vi "ML AI Player.vi"(0 "Total Player number":i32, 1 "Current Player ID number":i32, 2 "queue output":refnum<queue>, 3 "queue input":refnum<queue>) -> ()   [LabVIEW 2021]
uses:
  <vilib>/Utility/file.llb/Read Delimited Spreadsheet (DBL).vi
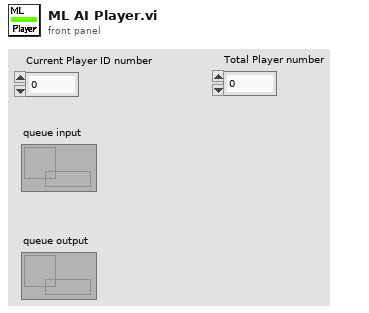
[diagram p1: front panel]
types:
  T1 = cluster{"all rows[1]":dbl, "all rows[2]":dbl, "all rows[3]":dbl, "all rows[4]":dbl, "all rows[5]":dbl, "all rows[6]":dbl, "all rows[7]":dbl, "all rows[8]":dbl, "all rows[9]":dbl}[]
  T2 = cluster{"X":dbl, "Y":dbl, "Object type":dbl, "Radius":dbl, "Width":dbl, "Height":dbl, "Theta":dbl, "HP":dbl, "R":dbl, "G":dbl, "B":dbl}[]
  T3 = cluster{"all rows[0]":dbl, "all rows[1]":dbl, "all rows[2]":dbl, "all rows[3]":dbl, "all rows[4]":dbl, "all rows[5]":dbl, "all rows[6]":dbl, "all rows[7]":dbl, "all rows[8]":dbl, "all rows[9]":dbl}
  T4 = cluster{"all rows[1]":dbl, "all rows[2]":dbl, "all rows[3]":dbl, "all rows[4]":dbl, "all rows[5]":dbl, "all rows[6]":dbl, "all rows[7]":dbl, "all rows[8]":dbl, "all rows[9]":dbl}
  T5 = cluster{"X":dbl, "Y":dbl, "Object type":dbl, "Radius":dbl, "Width":dbl, "Height":dbl, "Theta":dbl, "HP":dbl, "R":dbl, "G":dbl, "B":dbl}
  T6 = cluster{"D1":dbl, "D2":dbl, "D3":dbl, "D4":dbl, "D5":dbl, "D6":dbl, "D7":dbl, "D8":dbl}
  T7 = cluster{"Theta (toward that target)":dbl, "Distance (toward that target)":dbl, "Reachable":bool}
  T8 = cluster{dbl, dbl, "y":dbl, "y":dbl, "y":dbl, "y":dbl}
  T9 = cluster{dbl, dbl, "Theta (toward that target)":dbl, "f":dbl}
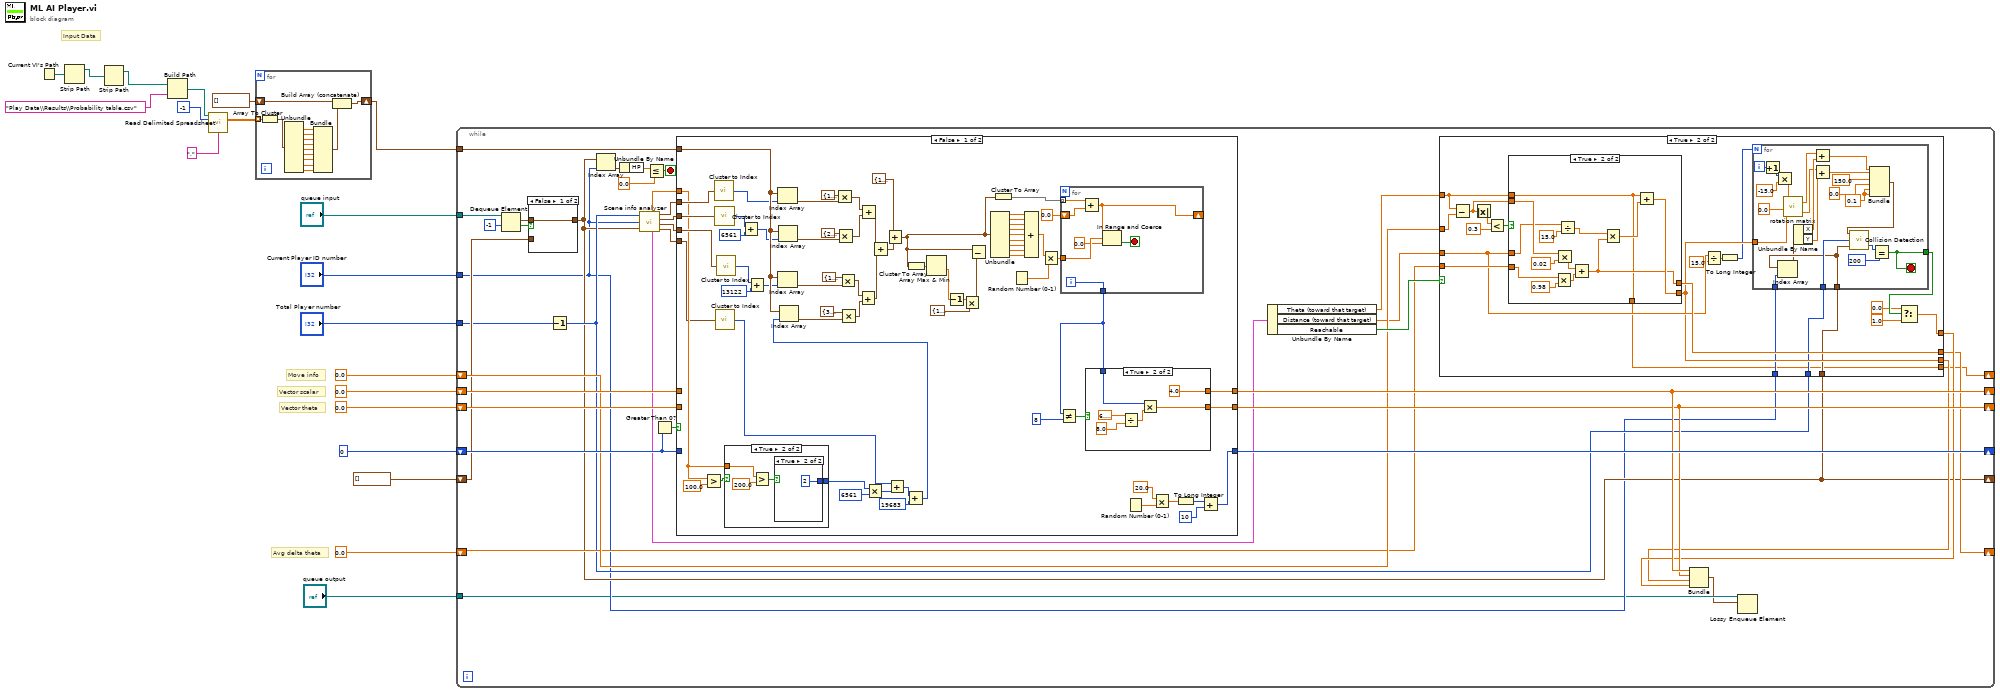
[diagram p0: block diagram]
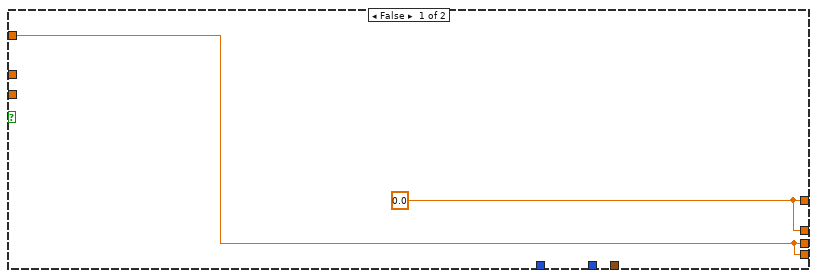
[diagram p3: hidden frame]
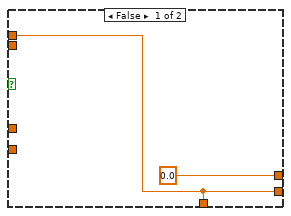
[diagram p4: hidden frame]
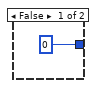
[diagram p5: hidden frame]
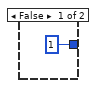
[diagram p6: hidden frame]
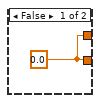
[diagram p7: hidden frame]
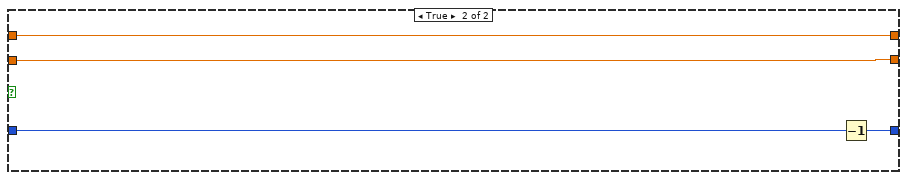
[diagram p8: hidden frame]
diagram:
  # "Input Data"
  # "Avg delta theta"
  # "Vector theta"
  # "Vector scalar"
  # "Move info"
  n1 = Current VI's Path() -> (path=w7:path)
  n2 = Strip Path(path=w7) -> (stripped path=w6:path)  [unwired: 1 out]
  n3 = Strip Path(path=w6) -> (stripped path=w5:path)  [unwired: 1 out]
  n4 = Build Path(base path=w5, name or relative path="Play Data\\Results\\Probability table.csv" ("delimiter (\\t)")) -> (appended path=w10:path)
  n5 = call-poly <vilib>:"Read Delimited Spreadsheet.vi"("file path (dialog if empty)"=w10, "number of rows (all:-1)"=-1, "delimiter (\\t)"="," ("delimiter (\\t)")) -> ("all rows"=w3:dbl[][])  [unwired: 7 in, 5 out]
  n6 = for {
    tunnel: w3 -> [w34] mode=indexing
    shift-right: [w33] -> w2
    shift-left: T1 [] -> [w32]
    n7 = Array To Cluster(array=w34) -> (cluster=w31:T3)
    n8 = Unbundle(w31) -> ("all rows[1]"=w30:dbl, "all rows[2]"=w29:dbl, "all rows[3]"=w28:dbl, "all rows[4]"=w27:dbl, "all rows[5]"=w26:dbl, "all rows[6]"=w25:dbl, "all rows[7]"=w24:dbl, "all rows[8]"=w23:dbl, "all rows[9]"=w22:dbl)  [unwired: 1 out]
    n9 = Bundle("all rows[1]"=w30, "all rows[2]"=w29, "all rows[3]"=w28, "all rows[4]"=w27, "all rows[5]"=w26, "all rows[6]"=w25, "all rows[7]"=w24, "all rows[8]"=w23, "all rows[9]"=w22) -> (w21:T4)  [unwired: 1 in]
    n10 = Build Array (concatenate)(w32, w21) -> (w33:T1)
  }
  n11 = while {
    tunnel: "queue input" -> [w41]
    shift-right: [w72] -> _
    shift-left: 0 -> [w70]
    tunnel: "queue output" -> [w37]
    shift-right: [w46] -> _
    shift-left: 0.0 -> [w58]
    shift-right: [w62] -> _
    shift-left: 0.0 -> [w64]
    shift-right: [w61] -> _
    shift-left: 0.0 -> [w63]
    shift-right: [w52] -> _
    shift-left: 0.0 -> [w53]
    shift-right: [w45] -> _
    shift-left: T2 [] ("Map Entity Object Position") -> [w44]
    tunnel: "Current Player ID number" -> [w43]
    tunnel: "Total Player number" -> [w42]
    tunnel: w2 -> [w35]
    stop <- w48 stop-if-true
    n12 = Dequeue Element(queue=w41, timeout in ms (-1)=-1) -> (element=w40:T2, timed out?=w38:bool)  [unwired: 1 in, 2 out]
    n13 = case shown="False" w38 {
      tunnel: [w73 w74] -> w45
      tunnel: w40 -> [w73 _]
      tunnel: w44 -> [_ w74]
      frame False {
      }
      frame True {
      }
    }
    n14 = Decrement(x=w42) -> (x-1=w51:i32)
    n15 = Index Array(array=w45, index=w43) -> (element=w50:T5)
    n16 = Unbundle By Name(w50) -> ("HP"=w49:dbl)
    n17 = call "Scene info analyzer.vi"("Map Entity Object Position"=w45, "Current Player ID"=w43, "Max Player ID"=w51) -> ("Enemy on 8 directions"=w65:T6, "Closest valid target"=w60:T7, "Farther Bullets on 8 directions"=w66:T6, "Closer Bullets on 8 directions"=w67:T6, "Current Player HP"=w69:dbl, "Object on 8 directions"=w68:T6)
    n18 = Less Or Equal?(x=w49, y=0.0) -> (x <= y?=w48:bool)
    n19 = Greater Than 0?(x=w70) -> (x > 0?=w71:bool)
    n20 = case shown="False" w71 {
      tunnel: [w203 w228] -> w72
      tunnel: w70 -> [_ w229]
      tunnel: w69 -> [w140 _]
      tunnel: w68 -> [w149 _]
      tunnel: w67 -> [w155 _]
      tunnel: w66 -> [w148 _]
      tunnel: w65 -> [w138 _]
      tunnel: w64 -> [_ w227]
      tunnel: w63 -> [_ w226]
      tunnel: [w204 w226] -> w61
      tunnel: [w166 w227] -> w62
      tunnel: w35 -> [w157 _]
      frame False {
        n21 = Greater?(x=w140, y=100.0) -> (0:w141:bool)
        n22 = call "Cluster to Index.vi"("Object on 8 directions"=w149) -> ("Index"=w156:i32)
        n23 = call "Cluster to Index.vi"("Object on 8 directions"=w155) -> ("Index"=w154:i32)
        n24 = call "Cluster to Index.vi"("Object on 8 directions"=w138) -> ("Index"=w137:i32)
        n25 = call "Cluster to Index.vi"("Object on 8 directions"=w148) -> ("Index"=w147:i32)
        n26 = case shown="True" w141 {
          tunnel: w140 -> [_ w207]
          tunnel: [0 ("y") w206] -> w139
          frame False {
          }
          frame True {
            n27 = Greater?(x=w207, y=200.0) -> (0:w208:bool)
            n28 = case shown="True" w208 {
              tunnel: [1 ("y") 2 ("y")] -> w206
              frame False {
              }
              frame True {
              }
            }
          }
        }
        n29 = Add(x=w154, y=6561) -> (x+y=w151:i32)
        n30 = Add(x=w147, y=13122) -> (x+y=w150:i32)
        n31 = Index Array(array=w157, index=w156) -> (element=w178:T4)
        n32 = Index Array(array=w157, index=w150) -> (element=w158:T4)
        n33 = Index Array(array=w157, index=w151) -> (element=w160:T4)
        n34 = Multiply(x=T4 {"all rows[1]"=1.5, "all rows[2]"=1.5, "all rows[3]"=1.5, "all rows[4]"=1.5, "all rows[5]"=1.5, "all rows[6]"=1.5, "all rows[7]"=1.5, "all rows[8]"=1.5, "all rows[9]"=1.5}, y=w178) -> (x*y=w179:T4)
        n35 = Multiply(x=T4 {"all rows[1]"=2.0, "all rows[2]"=2.0, "all rows[3]"=2.0, "all rows[4]"=2.0, "all rows[5]"=2.0, "all rows[6]"=2.0, "all rows[7]"=2.0, "all rows[8]"=2.0, "all rows[9]"=2.0}, y=w160) -> (x*y=w202:T4)
        n36 = Multiply(x=T4 {"all rows[1]"=1.5, "all rows[2]"=1.5, "all rows[3]"=1.5, "all rows[4]"=1.5, "all rows[5]"=1.5, "all rows[6]"=1.5, "all rows[7]"=1.5, "all rows[8]"=1.5, "all rows[9]"=1.5}, y=w158) -> (x*y=w201:T4)
        n37 = Add(x=w179, y=w202) -> (x+y=w199:T4)
        n38 = Multiply(x=w139, y=6561) -> (x*y=w143:i32)
        n39 = Add(x=w137, y=w143) -> (x+y=w145:i32)
        n40 = Add(x=w145, y=19683) -> (x+y=w136:i32)
        n41 = Index Array(array=w157, index=w136) -> (element=w159:T4)
        n42 = Multiply(x=T4 {"all rows[1]"=3.0, "all rows[2]"=3.0, "all rows[3]"=3.0, "all rows[4]"=3.0, "all rows[5]"=3.0, "all rows[6]"=3.0, "all rows[7]"=3.0, "all rows[8]"=3.0, "all rows[9]"=3.0}, y=w159) -> (x*y=w200:T4)
        n43 = Add(x=w201, y=w200) -> (x+y=w198:T4)
        n44 = Add(x=w199, y=w198) -> (x+y=w162:T4)
        n45 = Add(x=T4 {"all rows[1]"=1.0, "all rows[2]"=1.0, "all rows[3]"=1.0, "all rows[4]"=1.0, "all rows[5]"=1.0, "all rows[6]"=1.0, "all rows[7]"=1.0, "all rows[8]"=1.0, "all rows[9]"=1.0}, y=w162) -> (x+y=w161:T4)
        n46 = Cluster To Array(cluster=w161) -> (array=w172:dbl[])
        n47 = Array Max & Min(array=w172) -> (min value=w165:dbl)  [unwired: 3 out]
        n48 = Decrement(x=w165) -> (x-1=w164:dbl)
        n49 = Multiply(x=w164, y=T4 {"all rows[1]"=1.0, "all rows[2]"=1.0, "all rows[3]"=1.0, "all rows[4]"=1.0, "all rows[5]"=1.0, "all rows[6]"=1.0, "all rows[7]"=1.0, "all rows[8]"=1.0, "all rows[9]"=1.0} ("x")) -> (x*y=w170:T4)
        n50 = Subtract(x=w161, y=w170) -> ()  [unwired: 1 out]
        n51 = Unbundle(w161) -> ("all rows[1]"=w197:dbl, "all rows[2]"=w196:dbl, "all rows[3]"=w195:dbl, "all rows[4]"=w194:dbl, "all rows[5]"=w193:dbl, "all rows[6]"=w192:dbl, "all rows[7]"=w191:dbl, "all rows[8]"=w190:dbl, "all rows[9]"=w173:dbl)
        n52 = Cluster To Array(cluster=w161) -> (array=w187:dbl[])
        n53 = Random Number (0-1)() -> (number: 0 to 1=w189:dbl)
        n54 = Compound Arithmetic op=ADD(w197, w196, w195, w194, w193, w192, w191, w190, w173) -> (w188:dbl)
        n55 = Multiply(x=w188, y=w189) -> (x*y=w185:dbl)
        n56 = for {
          tunnel: w187 -> [w224] mode=indexing
          shift-right: [w223] -> _
          shift-left: 0.0 -> [w225]
          tunnel: w185 -> [w222]
          tunnel: [w221] -> w168
          i -> [w221]
          stop <- w220 stop-if-true
          n57 = Add(x=w224, y=w225) -> (x+y=w223:dbl)
          n58 = In Range and Coerce(upper limit=w223, x=w222, lower limit=0.0) -> (In Range?=w220:bool)  [unwired: 1 out]
        }
        n59 = Not Equal?(x=w168, y=8) -> (x != y?=w167:bool)
        n60 = case shown="True" w167 {
          tunnel: [w212 w218] -> w204
          tunnel: w168 -> [_ w214]
          tunnel: [w212 4.0] -> w166
          frame False {
            w212 = 0.0
          }
          frame True {
            n61 = Divide(x=6.283185307179586, y=8.0) -> (x/y=w215:dbl)
            n62 = Multiply(x=w214, y=w215) -> (x*y=w218:dbl)
          }
        }
        n63 = Random Number (0-1)() -> (number: 0 to 1=w183:dbl)
        n64 = Multiply(x=20.0, y=w183) -> (x*y=w182:dbl)
        n65 = To Long Integer(number=w182) -> (32bit integer=w180:i32)
        n66 = Add(x=w180, y=10) -> (x+y=w203:i32)
      }
      frame True {
        n67 = Decrement(x=w229) -> (x-1=w228:i32)
      }
    }
    n68 = Unbundle By Name(w60) -> ("Theta (toward that target)"=w55:dbl, "Distance (toward that target)"=w54:dbl, "Reachable"=w59:bool)
    n69 = case shown="True" w59 {
      tunnel: w58 -> [w75 w97]
      tunnel: [w75 w86] -> w56
      tunnel: [w76 w81] -> w57
      tunnel: w55 -> [_ w93]
      tunnel: w54 -> [_ w89]
      tunnel: w53 -> [_ w90]
      tunnel: [w76 w92] -> w52
      tunnel: w45 -> [_ w85]
      tunnel: w51 -> [_ w80]
      tunnel: w43 -> [_ w79]
      tunnel: [w75 w78] -> w46
      frame False {
        w76 = 0.0
      }
      frame True {
        n70 = Subtract(x=w93, y=w97) -> (x-y=w91:dbl)
        n71 = Absolute Value(x=w91) -> (abs(x)=w95:dbl)
        n72 = Less?(x=w95, y=0.3) -> (x < y?=w96:bool)
        n73 = case shown="True" w96 {
          tunnel: [w121 w131] -> w86
          tunnel: w93 -> [w121 w124]
          tunnel: [0.0 w126] -> w92
          tunnel: w90 -> [_ w129]
          tunnel: w91 -> [_ w130]
          tunnel: w89 -> [_ w127]
          tunnel: [w121 w124] -> w78
          frame False {
          }
          frame True {
            n74 = Multiply(x=w129, y=0.98) -> (x*y=w135:dbl)
            n75 = Multiply(x=w130, y=0.02) -> (x*y=w132:dbl)
            n76 = Divide(x=w127, y=15.0) -> (x/y=w123:dbl)
            n77 = Add(x=w132, y=w135) -> (x+y=w126:dbl)
            n78 = Multiply(x=w123, y=w126) -> (x*y=w125:dbl)
            n79 = Add(x=w124, y=w125) -> (x+y=w131:dbl)
          }
        }
        n80 = Divide(x=w89, y=15.0) -> (x/y=w87:dbl)
        n81 = To Long Integer(number=w87) -> (32bit integer=w77:i32)
        n82 = for {
          N: w77 -> [_]
          tunnel: w86 -> [w120]
          tunnel: w85 -> [w110]
          tunnel: [w98] -> w84
          tunnel: w80 -> [w116]
          tunnel: w79 -> [w111]
          i -> [w114]
          stop <- w98 stop-if-true
          w108 = 0.1 ("y")
          n83 = Increment(x=w114) -> (x+1=w113:i32)
          n84 = Multiply(x=w113, y=-15.0) -> (x*y=w112:dbl)
          n85 = Index Array(array=w110, index=w111) -> (element=w109:T5)
          n86 = call "rotation matrix.vi"("angle"=w120, "y"=0.0, "x"=w112) -> ("new y"=w102:dbl, "new x"=w101:dbl)
          n87 = Unbundle By Name(w109) -> ("X"=w103:dbl, "Y"=w104:dbl)
          n88 = Add(x=w101, y=w103) -> (x+y=w100:dbl)
          n89 = Add(x=w102, y=w104) -> (x+y=w99:dbl)
          n90 = Bundle(w100, w99, "y"=150.0, "y"=0.0, "y"=w108, "y"=w108) -> (w107:T8)  [unwired: 1 in]
          n91 = call "Collision Detection.vi"("Map Entity Objects Positions"=w110, "Max Player ID number"=w116, "Moving Object"=w107) -> ("Bullet hit Player No."=w118:i32)  [unwired: 1 out]
          n92 = Equal?(x=w118, y=200) -> (x = y?=w98:bool)
        }
        n93 = Select(t=0.0, s=w84, f=1.0) -> (s? t:f=w81:dbl)
      }
    }
    n94 = Bundle(w62, w61, "Theta (toward that target)"=w56, "f"=w57) -> (w36:T9)  [unwired: 1 in]
    n95 = Lossy Enqueue Element(queue=w37, element=w36) -> ()  [unwired: 1 in, 4 out]
  }
